vi "Testing PLC comm.vi"() -> ()   [LabVIEW 2017]
uses:
  Control/PLC_Comm_State.ctl
  <vilib>/DATA AHEAD/SP7/typedefs/PLC Type.ctl
  <vilib>/DATA AHEAD/SP7/typedefs/S7 Connection.ctl
  <vilib>/DATA AHEAD/SP7/functions/write/write Dint array.vi
  Global/DATA LOG.vi
  <vilib>/DATA AHEAD/SP7/functions/read/read Dint array.vi
  <vilib>/DATA AHEAD/SP7/functions/read/read String.vi
  <vilib>/DATA AHEAD/SP7/SP7.lvlib
panel:
  out "error out 3":errorcluster
  out "error out 2":errorcluster
  in  "stop":bool
  out "error out 4":errorcluster
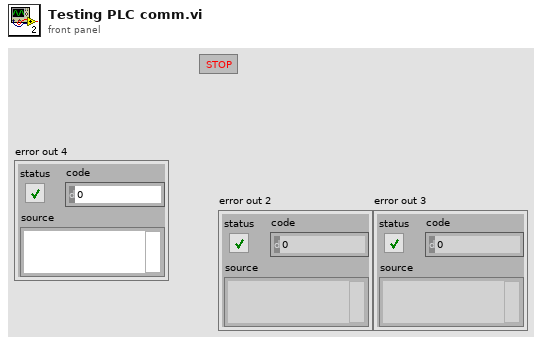
[diagram p1: front panel]
types:
  T1 = typedef "PLC_Comm_State.ctl" = enum16{"Int", "Connect", "Write", "Write2", "Write3", "Read", "Read2", "Read3", "Error", "Disconnect"}
  T2 = enum16{"Int", "Connect", "Write", "Read", "Error", "Disconnect"}
  T3 = typedef "SP7.lvlib/PLC Type.ctl" = enum16{"S7 200", "S7 300/400", "S7 1200", "S7 1500", "LOGO!8"}
  T4 = typedef "SP7.lvlib/S7 Connection.ctl" = cluster{"TCP Connection Ref":refnum<k5>, "IP address":string, "timeout ms":i32, "Connected?":bool, "PLC Type":T3, "Rack S7 400":u8, "Slot S7 400":u8, "PDU Size":u16, "connection semaphore":T5}
  T5 = typedef "Semaphore RefNum" = refnum<k1>
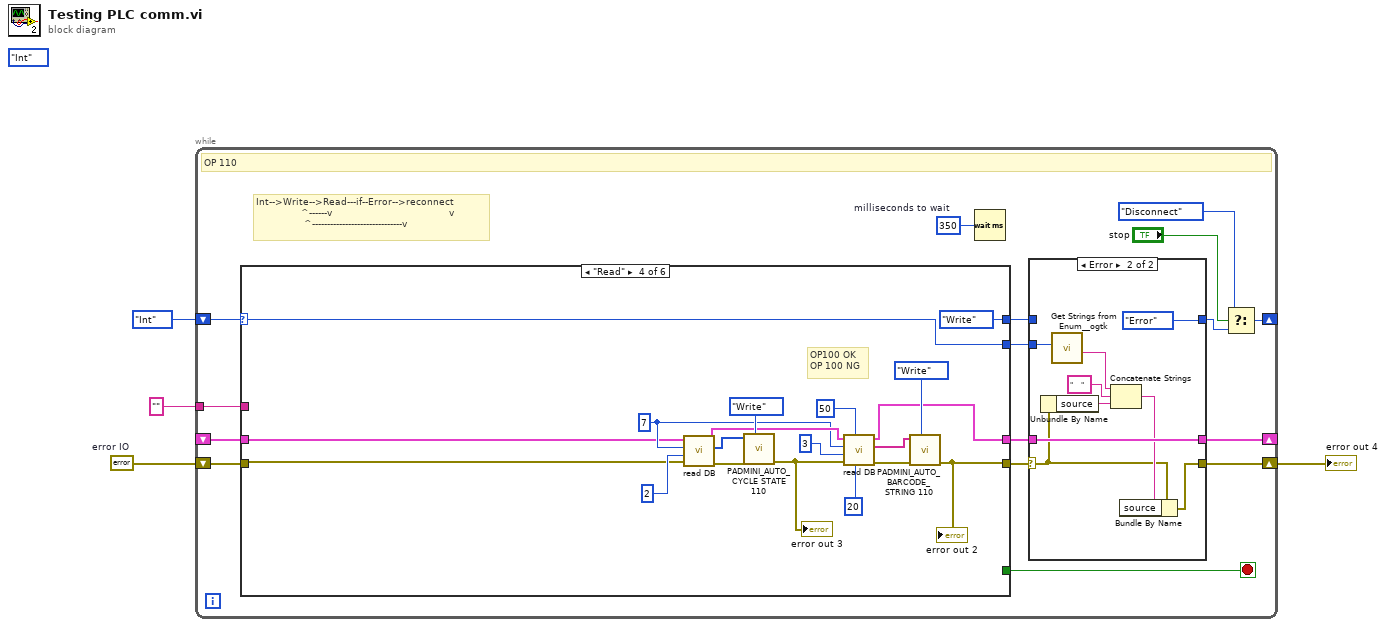
[diagram p0: block diagram]
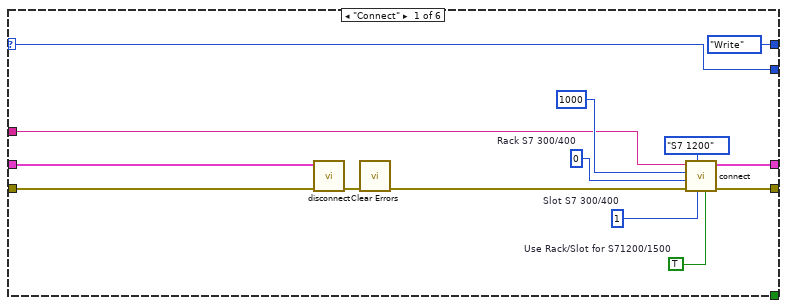
[diagram p3: hidden frame]
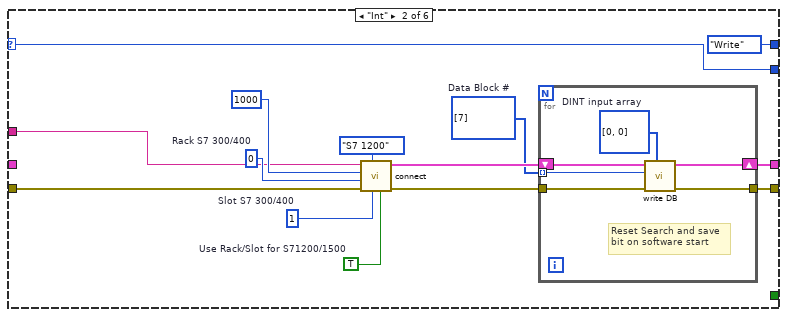
[diagram p4: hidden frame]
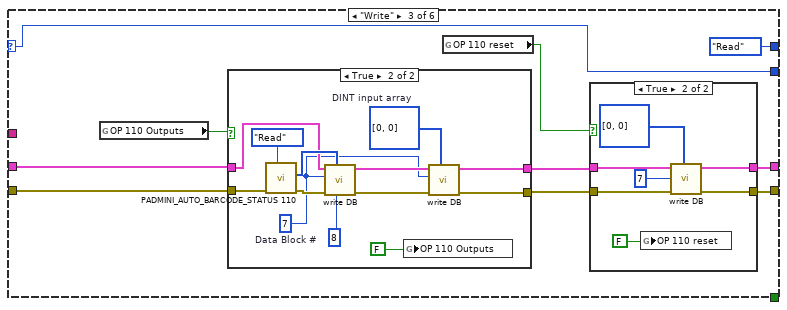
[diagram p5: hidden frame]
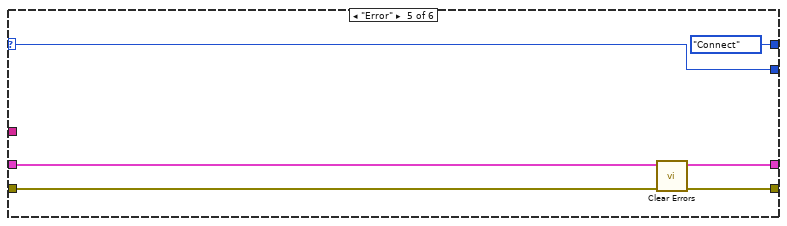
[diagram p8: hidden frame]
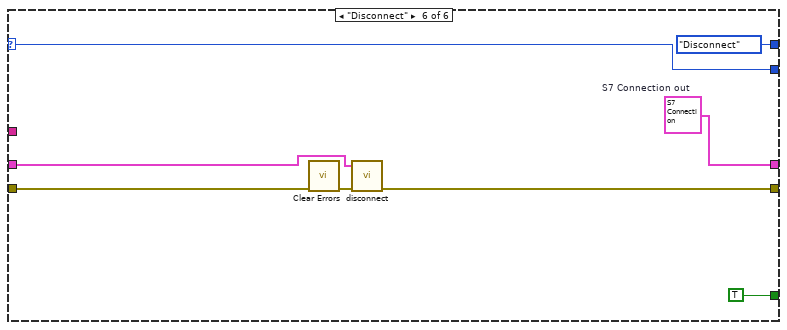
[diagram p9: hidden frame]
diagram:
  (unwired) PLC_Comm_State."Int"
  w1 = errorcluster {"status"=FALSE, "code"=0, "source"=""}  # error IO
  n1 = while {
    shift-right: [w9] -> _
    shift-left: T2."Int" -> [w19]
    shift-right: [w14] -> w4
    shift-left: w1 -> [w18]
    shift-right: [w12] -> _
    shift-left: _ -> [w17]
    tunnel: "" -> [w16]
    stop <- w10 stop-if-true
    w15 = u32 350  # milliseconds to wait
    # "Int-->Write-->Read---if--Error-->reconnect\n               ^------v                                       v\n                ^------------------------------v"
    # "OP 110"
    n2 = case shown="\"Read\"" w19 {
      selector: w19 -> [w33 w47 w67 w101 w120 w125]
      tunnel: [w39 w52 w72 w106 w122 w131] -> w20
      tunnel: [w40 w51 w71 w105 w124 w128] -> w11
      tunnel: w18 -> [w36 w50 w69 w103 w121 w129]
      tunnel: w17 -> [w34 _ w70 w104 w124 w130]
      tunnel: w16 -> [w41 w49 _ _ _ _]
      tunnel: [T2."Write" T2."Write" T2."Read" T2."Write" T2."Connect" T2."Disconnect"] -> w13
      tunnel: [_ _ _ _ _ TRUE] -> w10
      tunnel: [w33 w47 w67 w101 w120 w125] -> w5
      frame "Connect" {
        w46 = TRUE  # Use Rack/Slot for S71200/1500
        w45 = u8 1  # Slot S7 300/400
        w43 = u8 0  # Rack S7 300/400
        n3 = call <vilib>:"disconnect.vi"("error in (no error)"=w36, "S7 Connection in"=w34) -> ("error out"=w37:errorcluster)  [unwired: 8 in, 1 out]
        n4 = call <vilib>:"Clear Errors.vi"("error in (no error)"=w37) -> ("error out"=w35:errorcluster)  [unwired: 5 in, 1 out]
        n5 = call <vilib>:"connect.vi"("Use Rack/Slot for S71200/1500"=w46, "Slot S7 300/400"=w45, "PLC Type"=PLC_Type."S7 1200" ("PLC Type 2"), "error in (no error)"=w35, "Rack S7 300/400"=w43, "timeout [ms]"=1000 ("timeout [ms] 2"), "IP address"=w41) -> ("error out"=w39:errorcluster, "S7 Connection out"=w40:T4)  [unwired: 3 in]
      }
      frame "Int" {
        w53 = TRUE  # Use Rack/Slot for S71200/1500
        w54 = u8 1  # Slot S7 300/400
        w55 = u8 0  # Rack S7 300/400
        w56 = u16[] [7]  # Data Block #
        n6 = call <vilib>:"connect.vi"("Use Rack/Slot for S71200/1500"=w53, "Slot S7 300/400"=w54, "PLC Type"=PLC_Type."S7 1200" ("PLC Type 2"), "error in (no error)"=w50, "Rack S7 300/400"=w55, "timeout [ms]"=1000 ("timeout [ms] 2"), "IP address"=w49) -> ("error out"=w58:errorcluster, "S7 Connection out"=w57:T4)  [unwired: 3 in]
        n7 = for {
          tunnel: w56 -> [w66] mode=indexing
          shift-right: [w64] -> w51
          shift-left: w57 -> [w62]
          tunnel: w58 -> [w63]
          tunnel: [w61] -> w52
          w65 = i32[] [0, 0]  # DINT input array
          # "Reset Search and save \nbit on software start"
          n8 = call-poly <vilib>:"write DB.vi"("DINT input array"=w65, "error in (no error)"=w63, "Data Block #"=w66, "S7 Connection in"=w62) -> ("error out"=w61:errorcluster, "S7 Connection out"=w64:T4)  [unwired: 4 in, 2 out]
        }
      }
      frame "Write" {
        n9 = global read "DATA LOG.vi" "OP 110 Outputs"() -> (w76:bool)
        n10 = case shown="True" w76 {
          tunnel: [w86 w91] -> w75
          tunnel: [w87 w92] -> w74
          tunnel: w69 -> [w86 w96]
          tunnel: w70 -> [w87 w95]
          frame False {
          }
          frame True {
            w88 = i32[] [0, 0]  # DINT input array
            w89 = u16 7  # Data Block #
            n11 = call "PADMINI_AUTO_BARCODE_STATUS 110.vi"("Enum"=enum16{"Read", "Write"}."Read", "error in (no error)"=w96) -> ("error out"=w98:errorcluster, "O/P"=w99:i32[])  [unwired: 8 in]
            n12 = call-poly <vilib>:"write DB.vi"("Item offset [byte]"=u32 8, "DINT input array"=w99, "error in (no error)"=w98, "Data Block #"=w89, "S7 Connection in"=w95) -> ("error out"=w90:errorcluster, "S7 Connection out"=w93:T4)  [unwired: 3 in, 2 out]
            n13 = global write "DATA LOG.vi" "OP 110 Outputs"(FALSE) -> ()
            n14 = call-poly <vilib>:"write DB.vi"("DINT input array"=w88, "error in (no error)"=w90, "Data Block #"=w89, "S7 Connection in"=w93) -> ("error out"=w91:errorcluster, "S7 Connection out"=w92:T4)  [unwired: 4 in, 2 out]
          }
        }
        n15 = global read "DATA LOG.vi" "OP 110 reset"() -> (w73:bool)
        n16 = case shown="True" w73 {
          tunnel: w75 -> [w77 w85]
          tunnel: [w77 w84] -> w72
          tunnel: w74 -> [w78 w83]
          tunnel: [w78 w82] -> w71
          frame False {
          }
          frame True {
            n17 = global write "DATA LOG.vi" "OP 110 reset"(FALSE) -> ()
            n18 = call-poly <vilib>:"write DB.vi"("DINT input array"=i32[] [0, 0], "error in (no error)"=w85, "Data Block #"=u16 7, "S7 Connection in"=w83) -> ("error out"=w84:errorcluster, "S7 Connection out"=w82:T4)  [unwired: 4 in, 2 out]
          }
        }
      }
      frame "Read" {
        w114 = u16 7 ("Data Block #")
        # "OP100 OK\nOP 100 NG"
        n19 = call-poly <vilib>:"read DB.vi"("error in (no error)"=w103, "items #"=u16 2 ("Items # [byte]"), "Data Block #"=w114, "S7 Connection in"=w104) -> ("error out"=w118:errorcluster, "DINT result array"=w116:i32[], "S7 Connection out"=w115:T4)  [unwired: 5 in]
        n20 = call "PADMINI_AUTO_CYCLE STATE 110.vi"("Enum"=enum16{"Read", "Write"}."Write", "error in (no error)"=w118, "Input"=w116) -> ("error out"=w107:errorcluster)  [unwired: 7 in, 1 out]
        "error out 3" <- w107
        n21 = call-poly <vilib>:"read DB.vi"("Item offset [byte]"=u32 20, "String length reserved in DB (default=254)"=u16 50, "error in (no error)"=w107, "items #"=u16 3 ("Items # [byte]"), "Data Block #"=w114, "S7 Connection in"=w115) -> ("error out"=w110:errorcluster, "STRING result Array"=w111:string[], "S7 Connection out"=w105:T4)  [unwired: 2 in, 1 out]
        n22 = call "PADMINI_AUTO_BARCODE_STRING 110.vi"("Enum"=enum16{"Read", "Write"}."Write", "error in (no error)"=w110, "Input"=w111) -> ("error out"=w106:errorcluster)  [unwired: 7 in, 1 out]
        "error out 2" <- w106
      }
      frame "Error" {
        n23 = call <vilib>:"Clear Errors.vi"("error in (no error)"=w121) -> ("error out"=w122:errorcluster)  [unwired: 5 in, 1 out]
      }
      frame "Disconnect" {
        w128 = T4 {"TCP Connection Ref"=refnum, "IP address"="", "timeout ms"=5000, "Connected?"=FALSE, "PLC Type"=enum."S7 1200", "Rack S7 400"=0, "Slot S7 400"=0, "PDU Size"=0, "connection semaphore"=refnum}  # S7 Connection out
        n24 = call <vilib>:"Clear Errors.vi"("error in (no error)"=w129) -> ("error out"=w132:errorcluster)  [unwired: 5 in, 1 out]
        n25 = call <vilib>:"disconnect.vi"("error in (no error)"=w132, "S7 Connection in"=w130) -> ("error out"=w131:errorcluster)  [unwired: 8 in, 1 out]
      }
    }
    n26 = Wait (ms)(milliseconds to wait=w15) -> ()  [unwired: 1 out]
    n27 = case shown="Error" w20 {
      selector: w20 -> [w23 w25]
      tunnel: [w23 w24] -> w14
      tunnel: [w22 T2."Error"] -> w8
      tunnel: w13 -> [w22 _]
      tunnel: [w21 w31] -> w12
      tunnel: w11 -> [w21 w31]
      tunnel: w5 -> [_ w29]
      frame No Error {
      }
      frame Error {
        n28 = Unbundle By Name(w25) -> ("source"=w30:string)
        n29 = call <userlib>:"Get Strings from Enum__ogtk.vi"("Enum"=w29) -> ("String Value"=w28:string)  [unwired: 7 in, 3 out]
        n30 = Concatenate Strings(w28, "    " ("string"), w30) -> (w26:string)
        n31 = Bundle By Name(cluster=w25, "source"=w26) -> (w24:errorcluster)
      }
    }
    n32 = Select(t=T2."Disconnect", s="stop", f=w8) -> (s? t:f=w9:T2)
  }
  "error out 4" <- w4
